vi "WriteScriptFile.vi"(8 "error in (no error)":errorcluster, 10 "Script":string[][](array[string]), 11 "Path":path) -> (0 "error out":errorcluster)   [LabVIEW 2011]
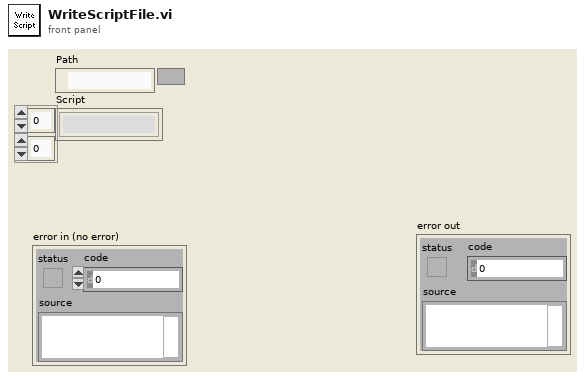
[diagram p1: front panel]
types:
  T1 = enum16{"open", "replace", "create", "open or create", "replace or create", "replace or create with confirmation"}
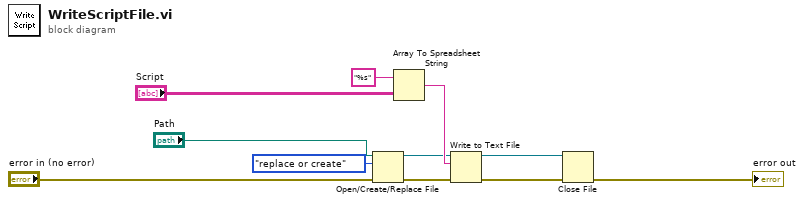
[diagram p0: block diagram]
diagram:
  n1 = Open/Create/Replace File(file path (use dialog)="Path", error in="error in (no error)", operation (0:open)=T1."replace or create") -> (refnum out=w4:refnum<file>, error out=w2:errorcluster)  [unwired: 4 out]
  n2 = Array To Spreadsheet String(array="Script", 3:"%s" ("format string")) -> (spreadsheet string=w11:string)  [unwired: 1 out]
  n3 = Write to Text File(file (use dialog)=w4, text=w11, error in=w2) -> (refnum out=w5:refnum<file>, error out=w3:errorcluster)  [unwired: 2 out]
  n4 = Close File(refnum=w5, error in=w3) -> (error out=→"error out":errorcluster)  [unwired: 1 out]
